vi "rm_empty_string.vi"(1 "Array":string[](array[string])) -> (0 "String output":string[](array[string]))   [LabVIEW 2017]
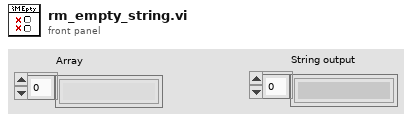
[diagram p1: front panel]
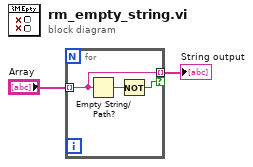
[diagram p0: block diagram]
diagram:
  n1 = for {
    tunnel: "Array" -> [w5] mode=indexing
    tunnel: [w5] -> w1 mode=indexing if=w3
    n2 = Empty String/Path?(string/path=w5) -> (empty?=w4:bool)
    n3 = Not(x=w4) -> (.not. x?=w3:bool)
  }
  "String output" <- w1
